vi "nanomsg_recv_timeout.vi"(4 "error in":errorcluster, 5 "timeout (ms)":u32=500, 6 "no block? (F)":bool, 7 "socket in":refnum<class "nanomsg_socket.lvclass">) -> (0 "error out":errorcluster, 1 "timeout?":bool, 2 "part":string, 3 "socket out":refnum<class "nanomsg_socket.lvclass">)   [LabVIEW 2014, in "nanomsg.lvlib" / "nanomsg_socket.lvclass"]
doc: "An implementation of \"receive with timeout\" functionality, returning an array of strings as per zmq_recv_multi. This VI is provided as a development \"crutch\" and is against the ZeroMQ philosophy but is highly convenient in some situations.\n\nPolls <b>socket in</b> periodically every <b>poll interval</b> milliseconds until a message has been received, or <b>timeout</b> milliseconds elapses since the start of the call. Aborts on error.\n\nDetailed API documentation: http://api.zeromq.org/3-2:zmq-poll"
uses:
  nanomsg_socket.lvclass
  nanomsg_socket.lvclass/nanomsg_socket.ctl
  <vilib>/Utility/error.llb/Error Cluster From Error Code.vi
  nanomsg.lvlib
panel:
  # "NN"
  # "labview"
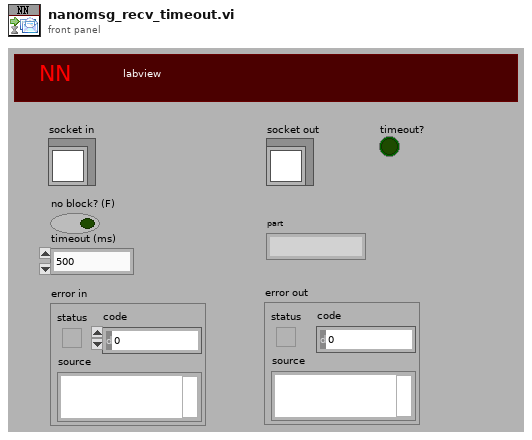
[diagram p1: front panel]
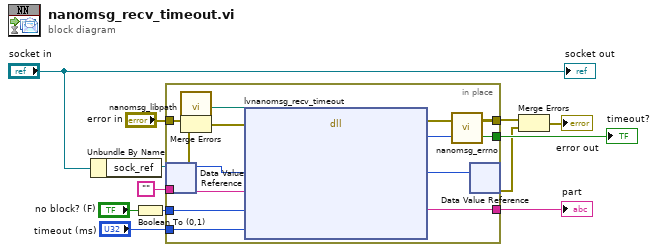
[diagram p0: block diagram]
diagram:
  n1 = Unbundle By Name("socket in") -> ("sock_ref"=w5:refnum<data-value>)
  n2 = Boolean To (0,1)(Boolean="no block? (F)") -> (0, 1=w1:i16)
  n3 = in-place {
    in-place-border: "" ("parts") -> [w26]
    in-place-border: [w25] -> w11
    in-place-border: "timeout (ms)" -> [w24]
    in-place-border: "error in" -> [w23]
    in-place-border: [w20] -> w8
    in-place-border: [w19] -> w7
    in-place-border: w1 -> [w13]
    n4 = in-place-dvr #1(w5) -> (w18:u64, w14:errorcluster)
    n5 = call "nanomsg_libpath.vi"() -> ("path"=w16:path)
    n6 = Merge Errors(w23, w14) -> (w15:errorcluster)
    n7 = dll-call lib="?" fn="lvnanomsg_recv_timeout" ("zmq_labview.dll:lvzmq_socket")(path in=w16, error in=w15, "sock_obj"=w18, "data"=w26, "flags"=w13, "timeout"=w24) -> (error out=w22:errorcluster, "return type"=w21:i32, "sock_obj"=w17:u64, "data"=w25:string)  [unwired: 5 in, 1 out]
    n8 = call "nanomsg_errno.vi"("retval"=w21, "error in"=w22) -> ("again?"=w19:bool, "error out"=w20:errorcluster)
    n9 = in-place-dvr #1(w17) -> (w3:errorcluster)  [unwired: 1 out]
  }
  "part" <- w11
  "timeout?" <- w7
  n10 = Merge Errors(w8, w3) -> (→"error out":errorcluster)
  "socket out" <- "socket in"
